vi "Feria.vi"(10 "Precio":i32, 11 "Suma":i32) -> (2 "Mensaje":string, 3 "Feria":i32)   [LabVIEW 2017]
doc: "SubVI que contiene la maquina de estados que hace el calculo del cambio y actualizacion de monedas en el Spreadsheet."
uses:
  Controls/Cambio.ctl
  Controls/Data.ctl
  Controls/Data_In.ctl
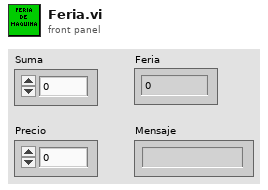
[diagram p1: front panel]
types:
  T1 = typedef "Data_In.ctl" = cluster{"Grand Total":i32, "Coca Cola":i32, "Pepsi":i32, "M5":i32, "M2":i32, "M1":i32}
  T2 = typedef "Data.ctl" = enum16{"Grand Total", "Coca-Cola", "Pepsi", "M1", "M2", "M5"}
  T3 = typedef "Cambio.ctl" = enum16{"M5", "M2", "M1", "Stop"}
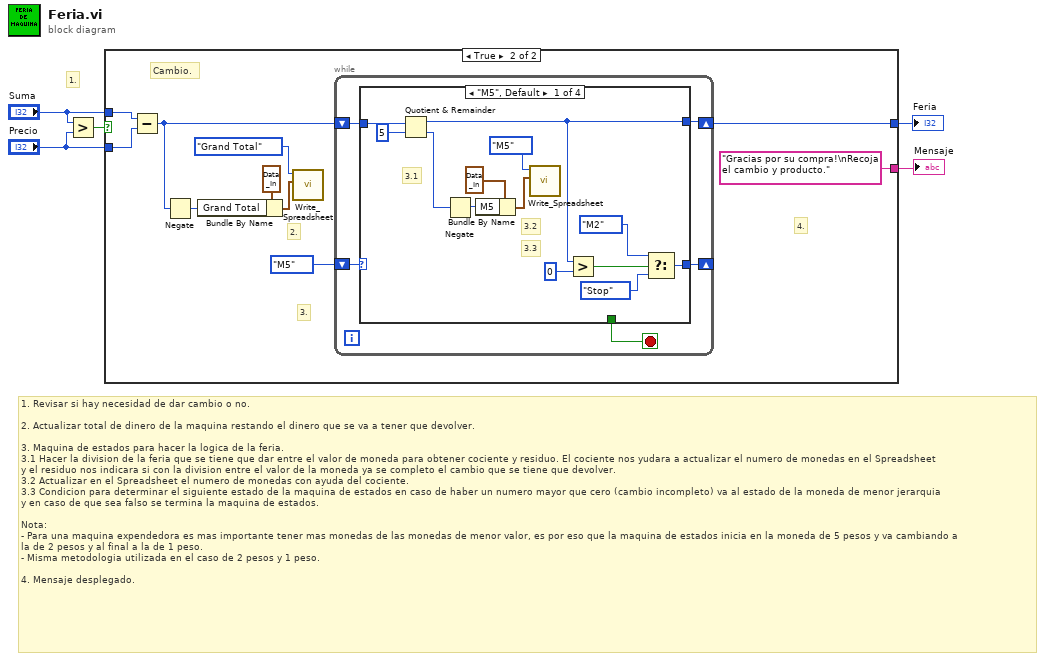
[diagram p0: block diagram]
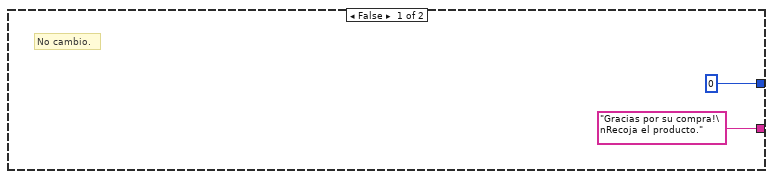
[diagram p2: hidden frame]
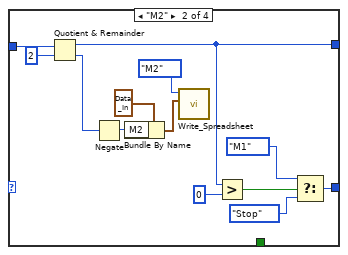
[diagram p3: hidden frame]
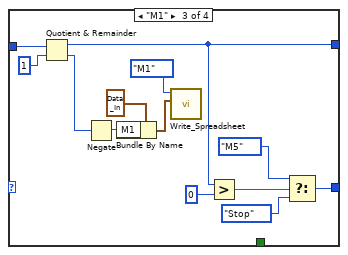
[diagram p4: hidden frame]
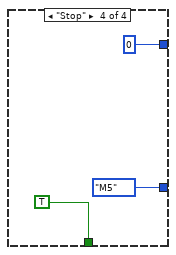
[diagram p5: hidden frame]
diagram:
  # "1. Revisar si hay necesidad de dar cambio o no.\n\n2. Actualizar total de dinero de la maquina restando el dinero que se va a tener que devolver.\n\n3. Maquina de estados para hacer la logica de la feria.\n3.1 Hacer la division de la feria que se tiene que dar entre el valor de moneda para obtener cociente y residuo. El cociente nos yudara a actualizar el numero de monedas en el Spreadsheet\ny el residuo nos indicara si con la division entre el valor de la moneda ya se completo el cambio que se tiene que devolver.\n3.2 Actualizar en el Spreadsheet el numero de monedas con ayuda del cociente.\n3.3 Condicion para determinar el siguiente estado de la maquina de estados en caso de haber un numero mayor que cero (cambio incompleto) va al estado de la moneda de menor jerarquia\ny en caso de que sea falso se termina la maquina de estados.\n\nNota:\n- Para una maquina expendedora es mas importante tener mas monedas de las monedas de menor valor, es por eso que la maquina de estados inicia en la moneda de 5 pesos y va cambiando a\nla de 2 pesos y al final a la de 1 peso.\n- Misma metodologia utilizada en el caso de 2 pesos y 1 peso.\n\n4. Mensaje desplegado."
  # "1."
  n1 = Greater?(x="Suma", y="Precio") -> (0:w5:bool)
  n2 = case shown="True" w5 {
    tunnel: "Suma" -> [_ w17]
    tunnel: "Precio" -> [_ w16]
    tunnel: [0 w14] -> w2
    tunnel: ["Gracias por su compra!\nRecoja el producto." "Gracias por su compra!\nRecoja el cambio y producto."] -> w1
    frame False {
      # "No cambio."
    }
    frame True {
      # "4."
      # "3."
      # "2."
      # "Cambio."
      n3 = Subtract(x=w17, y=w16) -> (x-y=w10:i32)
      n4 = Negate(x=w10) -> (-x=w12:i32)
      n5 = Bundle By Name(cluster=T1 {"Grand Total"=0, "Coca Cola"=0, "Pepsi"=0, "M5"=0, "M2"=0, "M1"=0} ("Data In"), "Grand Total"=w12) -> (w9:T1)
      n6 = call "Write_Spreadsheet.vi"("Data In"=w9, "Data"=Data."Grand Total") -> ()  [unwired: 10 in]
      n7 = while {
        shift-right: [w20] -> w14
        shift-left: w10 -> [w21]
        shift-right: [w18] -> _
        shift-left: Cambio."M5" ("Cambio") -> [w22]
        stop <- w19 stop-if-true
        n8 = case shown="\"M5\", Default" w22 {
          tunnel: w21 -> [w35 w48 w61 _]
          tunnel: [w27 w40 w53 0] -> w20
          tunnel: [_ _ _ TRUE] -> w19
          tunnel: [w23 w36 w49 Cambio."M5" ("Cambio")] -> w18
          frame "M5", Default {
            # "3.3"
            # "3.2"
            # "3.1"
            n9 = Quotient & Remainder(x=w35, y=5) -> (x-y*floor(x/y)=w27:i32, floor(x/y)=w29:i32)
            n10 = Negate(x=w29) -> (-x=w30:i32)
            n11 = Bundle By Name(cluster=T1 {"Grand Total"=0, "Coca Cola"=0, "Pepsi"=0, "M5"=0, "M2"=0, "M1"=0} ("Data In"), "M5"=w30) -> (w31:T1)
            n12 = call "Write_Spreadsheet.vi"("Data In"=w31, "Data"=Data."M5") -> ()  [unwired: 10 in]
            n13 = Greater?(x=w27, y=0) -> (0:w28:bool)
            n14 = Select(t=Cambio."M2" ("Cambio"), s=w28, f=Cambio."Stop" ("Cambio")) -> (s? t:f=w23:T3)
          }
          frame "M2" {
            n15 = Quotient & Remainder(x=w48, y=2) -> (x-y*floor(x/y)=w40:i32, floor(x/y)=w42:i32)
            n16 = Negate(x=w42) -> (-x=w43:i32)
            n17 = Bundle By Name(cluster=T1 {"Grand Total"=0, "Coca Cola"=0, "Pepsi"=0, "M5"=0, "M2"=0, "M1"=0} ("Data In"), "M2"=w43) -> (w44:T1)
            n18 = call "Write_Spreadsheet.vi"("Data In"=w44, "Data"=Data."M2") -> ()  [unwired: 10 in]
            n19 = Greater?(x=w40, y=0) -> (0:w41:bool)
            n20 = Select(t=Cambio."M1" ("Cambio"), s=w41, f=Cambio."Stop" ("Cambio")) -> (s? t:f=w36:T3)
          }
          frame "M1" {
            n21 = Quotient & Remainder(x=w61, y=1) -> (x-y*floor(x/y)=w53:i32, floor(x/y)=w55:i32)
            n22 = Negate(x=w55) -> (-x=w56:i32)
            n23 = Bundle By Name(cluster=T1 {"Grand Total"=0, "Coca Cola"=0, "Pepsi"=0, "M5"=0, "M2"=0, "M1"=0} ("Data In"), "M1"=w56) -> (w57:T1)
            n24 = call "Write_Spreadsheet.vi"("Data In"=w57, "Data"=Data."M1") -> ()  [unwired: 10 in]
            n25 = Greater?(x=w53, y=0) -> (0:w54:bool)
            n26 = Select(t=Cambio."M5" ("Cambio"), s=w54, f=Cambio."Stop" ("Cambio")) -> (s? t:f=w49:T3)
          }
          frame "Stop" {
          }
        }
      }
    }
  }
  "Feria" <- w2
  "Mensaje" <- w1
